vi "DEMO(MACRO).vi"() -> ()   [LabVIEW 2011]
panel:
  out "Output":string
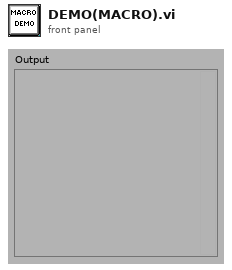
[diagram p1: front panel]
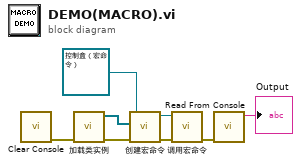
[diagram p0: block diagram]
diagram:
  n1 = call "Clear Console.vi"() -> ("error out"=w3:errorcluster)  [unwired: 11 in]
  n2 = call "加载类实例.vi"("error in (no error)"=w3) -> ("error out"=w2:errorcluster, "数组"=w1:refnum<class "命令类.lvclass">[])  [unwired: 9 in]
  n3 = call "创建宏命令.vi"("error in (no error)"=w2, "宏命令"=w1, "控制盒（宏命令） 输入"=refnum<class "控制盒（宏命令）.lvclass"> refnum ("控制盒（宏命令）.lvclass")) -> ("error out"=w6:errorcluster, "控制盒（宏命令） 输出"=w5:refnum<class "控制盒（宏命令）.lvclass">)  [unwired: 7 in]
  n4 = call "调用宏命令.vi"("error in (no error)"=w6, "控制盒（宏命令） 输入"=w5) -> ("error out"=w4:errorcluster)  [unwired: 8 in, 1 out]
  n5 = call "Read From Console.vi"("error in (no error)"=w4) -> ("Output"=→"Output":string)  [unwired: 9 in, 1 out]
